vi "XIPIN_Multiply_Accumulator_2_0.vi"   [LabVIEW 2017]
doc: "The Xilinx LogiCORE Multiply Accumulator generates a multiply accumulate function implemented in Xtreme DSP(TM) slices. User options allow you to specify the wordlengths of the inputs and the accumulation width.\n------------------------------------\n<b>Need License</b> : No"
uses:
  <vilib>/rvi/XilinxIP/XIPIN_XNode/niFpgaXIPIN.xnode
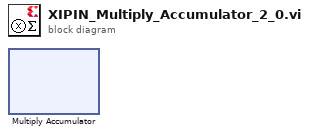
[diagram p0: block diagram]
diagram:
  n1 = xnode ("Multiply Accumulator")() -> ()
